vi "Combinations4Of60_all.vi"() -> ()   [LabVIEW 2019]
panel:
  in  "Numeric 2":i32=4
  in  "Numeric":i32=60
  out "size(s)":i32[](array[numeric])
  out "All possible permutations (4 of 60)":u8[][](array[numeric])
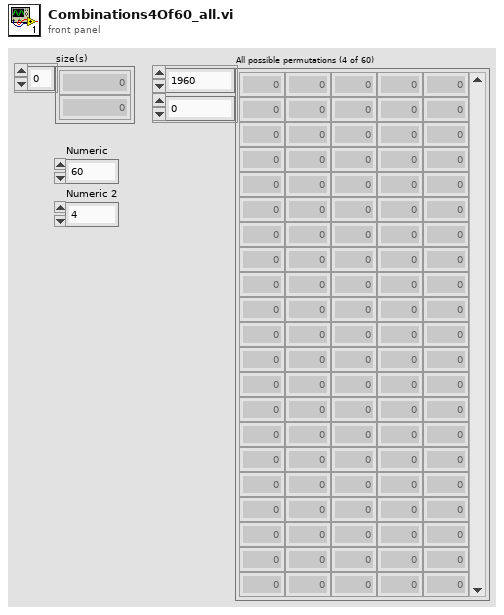
[diagram p1: front panel]
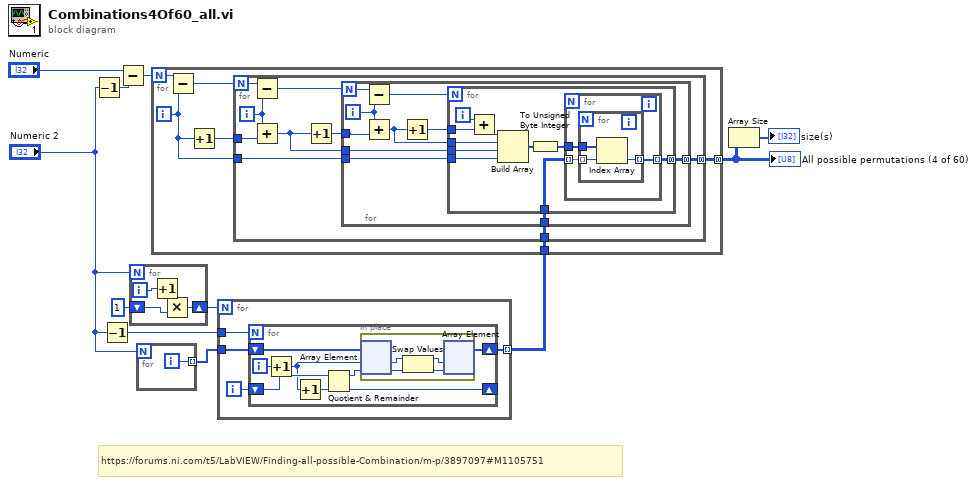
[diagram p0: block diagram]
diagram:
  # "https://forums.ni.com/t5/LabVIEW/Finding-all-possible-Combination/m-p/3897097#M1105751"
  n1 = Decrement(x="Numeric 2") -> (x-1=w10:i32)
  n2 = Decrement(x="Numeric 2") -> (x-1=w1:i32)
  n3 = Subtract(x="Numeric", y=w10) -> (x-y=w11:i32)
  n4 = for {
    N: "Numeric 2" -> [_]
    shift-right: [w14] -> w3
    shift-left: 1 -> [w12]
    i -> [w13]
    n5 = Increment(x=w13) -> (x+1=w15:i32)
    n6 = Multiply(x=w15, y=w12) -> (x*y=w14:i32)
  }
  n7 = for {
    N: "Numeric 2" -> [_]
    tunnel: [w16] -> w4 mode=indexing
    i -> [w16]
  }
  n8 = for {
    N: w3 -> [_]
    tunnel: w4 -> [w20]
    tunnel: [w18] -> w5 mode=indexing
    tunnel: w1 -> [w17]
    i -> [w19]
    n9 = for "loop over j (2..length(s))" {
      N: w17 -> [_]
      shift-right: [w21] -> w18
      shift-left: w20 -> [w22]
      shift-right: [w26] -> _
      shift-left: w19 -> [w28]
      i -> [w27]
      n10 = Increment(x=w27) -> (x+1=w24:i32)
      n11 = Increment(x=w24) -> (x+1=w25:i32)
      n12 = Quotient & Remainder(x=w28, y=w25) -> (x-y*floor(x/y)=w23:i32, floor(x/y)=w26:i32)
      n13 = in-place {
        n14 = in-place-array #1(w22, w24, w23) -> (w31:i32, w32:i32)
        n15 = Swap Values(12:w31, 14:w32) -> (1:w30:i32, 3:w29:i32)  [unwired: 1 in]
        n16 = in-place-array #1(w30, w29) -> (w21:i32[])  [unwired: 2 out]
      }
    }
  }
  n17 = for {
    N: w11 -> [w36]
    tunnel: [w35] -> w8 mode=concatenating
    tunnel: w5 -> [w33]
    i -> [w34]
    n18 = Subtract(x=w36, y=w34) -> (x-y=w38:i32)
    n19 = Increment(x=w34) -> (x+1=w37:i32)
    n20 = for {
      N: w38 -> [w47]
      tunnel: w37 -> [w43]
      tunnel: w34 -> [w42]
      tunnel: [w41] -> w35 mode=concatenating
      tunnel: w33 -> [w39]
      i -> [w44]
      n21 = Subtract(x=w47, y=w44) -> (x-y=w46:i32)
      n22 = Add(x=w44, y=w43) -> (x+y=w40:i32)
      n23 = Increment(x=w40) -> (x+1=w45:i32)
      n24 = for {
        N: w46 -> [w57]
        tunnel: w45 -> [w55]
        tunnel: w40 -> [w52]
        tunnel: w42 -> [w51]
        tunnel: [w50] -> w41 mode=concatenating
        tunnel: w39 -> [w48]
        i -> [w56]
        n25 = Subtract(x=w57, y=w56) -> (x-y=w53:i32)
        n26 = Add(x=w56, y=w55) -> (x+y=w49:i32)
        n27 = Increment(x=w49) -> (x+1=w54:i32)
        n28 = for {
          N: w53 -> [_]
          tunnel: w54 -> [w67]
          tunnel: w49 -> [w65]
          tunnel: w52 -> [w64]
          tunnel: w51 -> [w63]
          tunnel: [w60] -> w50 mode=concatenating
          tunnel: w48 -> [w59]
          i -> [w66]
          n29 = Add(x=w66, y=w67) -> (x+y=w62:i32)
          n30 = Build Array(w62, w65, w64, w63) -> (w61:i32[])
          n31 = To Unsigned Byte Integer(number=w61) -> (unsigned 8bit integer=w58:u8[])
          n32 = for {
            tunnel: w58 -> [w70]
            tunnel: [w68] -> w60 mode=indexing
            tunnel: w59 -> [w69] mode=indexing
            n33 = for {
              tunnel: w70 -> [w73]
              tunnel: w69 -> [w72] mode=indexing
              tunnel: [w71] -> w68 mode=indexing
              n34 = Index Array(array=w73, index=w72) -> (element=w71:u8)
            }
          }
        }
      }
    }
  }
  "All possible permutations (4 of 60)" <- w8
  n35 = Array Size(array=w8) -> (size(s)=→"size(s)":i32[])
